vi "Read PNG zTXt Chunk.vi"(10 "error in (no error)":errorcluster, 11 "data":u8[](array[numeric])) -> (2 "error out":errorcluster, 3 "String":string)   [LabVIEW 2021, in "Files.lvlib"]
uses:
  Files.lvlib
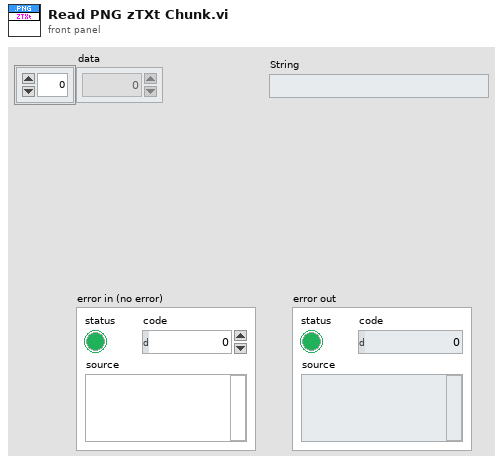
[diagram p1: front panel]
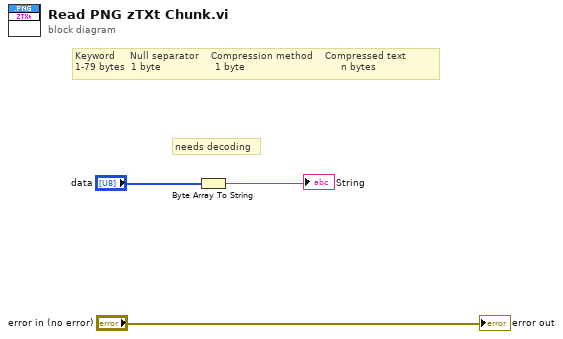
[diagram p0: block diagram]
diagram:
  # "Keyword \t   Null separator   \tCompression method \t  Compressed text\n1-79 bytes \t1 byte \t                1 byte                               \tn bytes"
  # "needs decoding"
  n1 = Byte Array To String(unsigned byte array="data") -> (string=→"String":string)
  "error out" <- "error in (no error)"
